vi "Break.vi"(8 "error in (no error)":errorcluster, 11 "Iterator NR Actor in":refnum<class "Iterator NR Actor.lvclass">) -> (0 "error out":errorcluster, 3 "Iterator NR Actor out":refnum<class "Iterator NR Actor.lvclass">)   [LabVIEW 2023, in "Iterator Actor.lvlib" / "Iterator NR Actor.lvclass"]
uses:
  Iterator NR Actor.lvclass
  Iterator NR Actor.lvclass/Iterator NR Actor.ctl
  <vilib>/ErrorRing/Error Ring.xnode
  <vilib>/Utility/error.llb/Error Cluster From Error Code.vi
  <vilib>/ActorFramework/Report Error Msg/Report Error Msg.lvclass
  <vilib>/ActorFramework/Actor/Actor.lvclass
  C:/Projects/Iterator Actor/Abstract Iterator Actor/Abstract Iterator Actor.lvclass
  C:/Program Files/National Instruments/LabVIEW 2023/vi.lib/LS Instruments AG/Async Methods Actor/Async Methods Actor/Async Methods Actor/Async Methods Actor.lvclass
  C:/Program Files/National Instruments/LabVIEW 2023/vi.lib/ActorFramework/Actor/Actor.lvclass
  C:/Projects/Iterator Actor/Iterator NR Actor/Iterator NR Actor Folder/Iterator NR Actor.lvclass
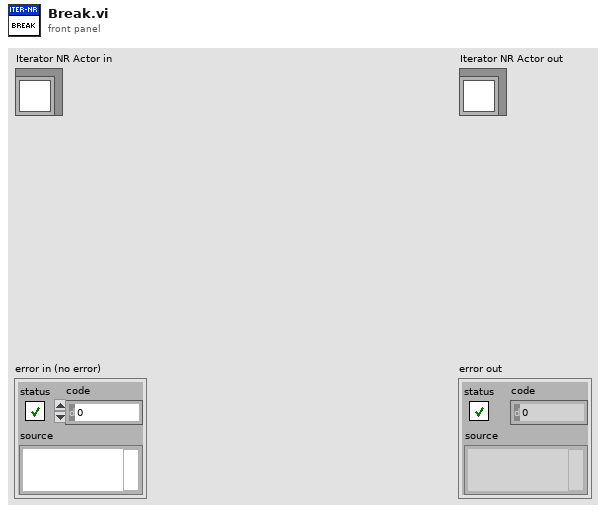
[diagram p1: front panel]
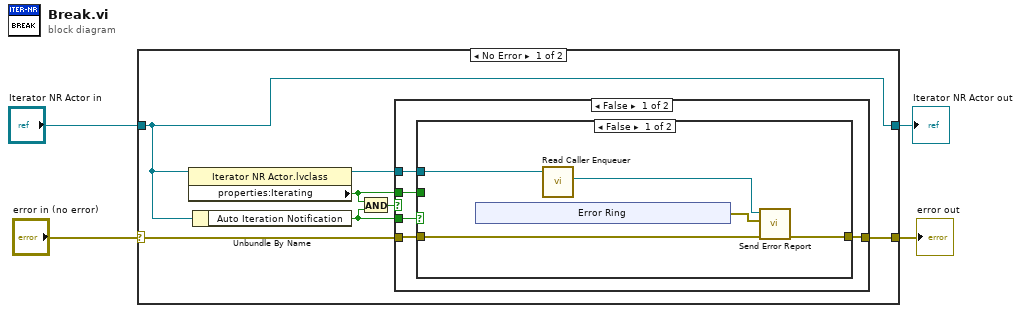
[diagram p0: block diagram]
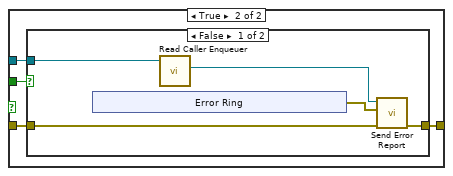
[diagram p2: hidden frame]
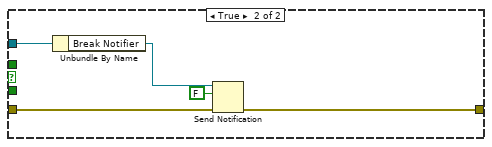
[diagram p4: hidden frame]
diagram:
  n1 = case shown="No Error" "error in (no error)" {
    selector: "error in (no error)" -> [w10 w46]
    tunnel: [w9 w46] -> w3
    tunnel: [w8 w45] -> w1
    tunnel: "Iterator NR Actor in" -> [w8 w45]
    frame No Error {
      n2 = property class="Iterator NR Actor.lvclass"(reference=w8) -> (reference out=w11:refnum<class "Iterator NR Actor.lvclass">, "properties:Iterating"=w5:bool)  [unwired: 1 in, 1 out]
      n3 = Unbundle By Name(w8) -> ("Auto Iteration Notification"=w6:bool)
      n4 = And(x=w5, y=w6) -> (x .and. y?=w7:bool)
      n5 = case shown="False" w7 {
        tunnel: w11 -> [w15 w44]
        tunnel: w10 -> [w13 w41]
        tunnel: [w14 w40] -> w9
        tunnel: w6 -> [w16 _]
        tunnel: w5 -> [w12 _]
        frame False {
          n6 = case shown="False" w16 {
            tunnel: w15 -> [w18 w26]
            tunnel: [w21 w28] -> w14
            tunnel: w13 -> [w20 w27]
            tunnel: w12 -> [_ w29]
            frame False {
              n7 = xnode "Error Ring"() -> ("error out"=w19:errorcluster)
              n8 = call <vilib>:"Read Caller Enqueuer.vi"("Actor"=w18) -> ("Caller Enqueuer"=w17:refnum<class "Message Enqueuer.lvclass">)  [unwired: 10 in]
              n9 = call <vilib>:"Send Error Report.vi"("error in (no error)"=w20, "Error From Sender"=w19, "Message Enqueuer"=w17) -> ("error out"=w21:errorcluster)  [unwired: 8 in]
            }
            frame True {
              n10 = case shown="False" w29 {
                tunnel: [w32 w39] -> w28
                tunnel: w27 -> [w31 w39]
                tunnel: w26 -> [w30 _]
                frame False {
                  n11 = xnode "Error Ring"() -> ("error out"=w34:errorcluster)
                  n12 = call <vilib>:"Read Caller Enqueuer.vi"("Actor"=w30) -> ("Caller Enqueuer"=w33:refnum<class "Message Enqueuer.lvclass">)  [unwired: 10 in]
                  n13 = call <vilib>:"Send Error Report.vi"("error in (no error)"=w31, "Error From Sender"=w34, "Message Enqueuer"=w33) -> ("error out"=w32:errorcluster)  [unwired: 8 in]
                }
                frame True {
                }
              }
            }
          }
        }
        frame True {
          n14 = Unbundle By Name(w44) -> ("Break Notifier"=w43:refnum<notifier>)
          n15 = Send Notification(notification=FALSE, notifier=w43, error in (no error)=w41) -> (error out=w40:errorcluster)  [unwired: 1 out]
        }
      }
    }
    frame Error {
    }
  }
  "error out" <- w3
  "Iterator NR Actor out" <- w1
